vi "uber auto.vi"(1 "autobox switches":cluster{bool, bool, bool}) -> ()   [LabVIEW 2011]
uses:
  <vilib>/Rock Robotics/WPI/Solenoid/WPI_SolenoidValue.ctl
  <vilib>/addons/control/pid/pid.llb/PID (DBL).vi
  <vilib>/Rock Robotics/WPI/Solenoid/WPI_SolenoidSetEnum.vi
  <vilib>/Rock Robotics/WPI/Solenoid/Deprecated/WPI_SolenoidSetBool.vi
  <vilib>/addons/control/pid/NI_PID_pid.lvlib
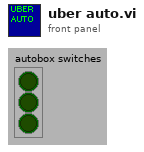
[diagram p1: front panel]
types:
  T1 = typedef "WPI_SolenoidDevRef.ctl" = cluster{"DevStatus":errorcluster, "Solenoid Module":T2, "Forward Solenoid Channel":T3, "Reverse Solenoid Channel":T3}
  T2 = typedef "FPGA_TypedefSolenoidModule.ctl" = enum16{"Solenoid Module 1", "Solenoid Module 2"}
  T3 = typedef "WPI_SolenoidChannel.ctl" = enum8{"Solenoid 1", "Solenoid 2", "Solenoid 3", "Solenoid 4", "Solenoid 5", "Solenoid 6", "Solenoid 7", "Solenoid 8", "Invalid"}
  T4 = typedef "WPI_EncoderDevRef.ctl" = cluster{"DevStatus":errorcluster, "EncoderIndex":T5, "CounterIndex":T6, "DistancePerCount":dbl, "Decoding Type":T7}
  T5 = typedef "FPGA_EncoderIdx.ctl" = enum8{"Enc 0", "Enc 1", "Enc 2", "Enc 3", "Invalid"}
  T6 = typedef "FPGA_CounterCtrSystemIndex.ctl" = enum8{"Ctr 0", "Ctr 1", "Ctr 2", "Ctr 3", "Ctr 4", "Ctr 5", "Ctr 6", "Ctr 7", "Invalid"}
  T7 = typedef "WPI_EncoderType.ctl" = enum16{"1x", "2x", "4x"}
  T8 = typedef "WPI_MotorControlDeviceRef.ctl" = cluster{"DeviceStatus":errorcluster, "Type":enum16{"PWM", "CAN"}, "PWM":cluster{"Digital Module":T9, "PWM Channel":T10, "DeadBand":T11}, "CAN":cluster{"Device Number":u8, "Control Mode":T12, "Semaphore":T13, "Max Vout":dbl}, "Invert":bool, "TransformRef":T14, "InvTransformRef":T14}
  T9 = typedef "FPGA_TypedefDigitalModule.ctl" = enum16{"Digital Module 1", "Digital Module 2"}
  T10 = typedef "FPGA_DIOPWMChannel.ctl" = enum8{"PWM 1", "PWM 2", "PWM 3", "PWM 4", "PWM 5", "PWM 6", "PWM 7", "PWM 8", "PWM 9", "PWM 10", "Invalid"}
  T11 = typedef "WPI_PWMDeadband.ctl" = cluster{"Name":string, "maxPositivePwm":i32, "minPositivePwm":i32, "centerPwm":i32, "maxNegativePwm":i32, "minNegativePwm":i32, "angularRange":u16}
  T12 = typedef "WPI_CANJaguar_ControlMode.ctl" = enum8{"Percent VBus", "Current", "Speed", "Position", "Voltage"}
  T13 = typedef "Semaphore RefNum" = refnum<k1>
  T14 = typedef "WPI_PWMTransform_ConPane.ctl" = refnum<vi>
  T15 = typedef "WPI_RobotDriveDevRef.ctl" = cluster{"DevStatus":errorcluster, "Motors[]":T8[], "Square Inputs":bool, "Max Output":dbl, "Isochronous":bool}
  T16 = cluster{"proportional gain (Kc)":dbl, "integral time (Ti, min)":dbl, "derivative time (Td, min)":dbl}
  T17 = typedef "WPI_SolenoidValue.ctl" = enum16{"Off", "On", "Forward", "Reverse"}
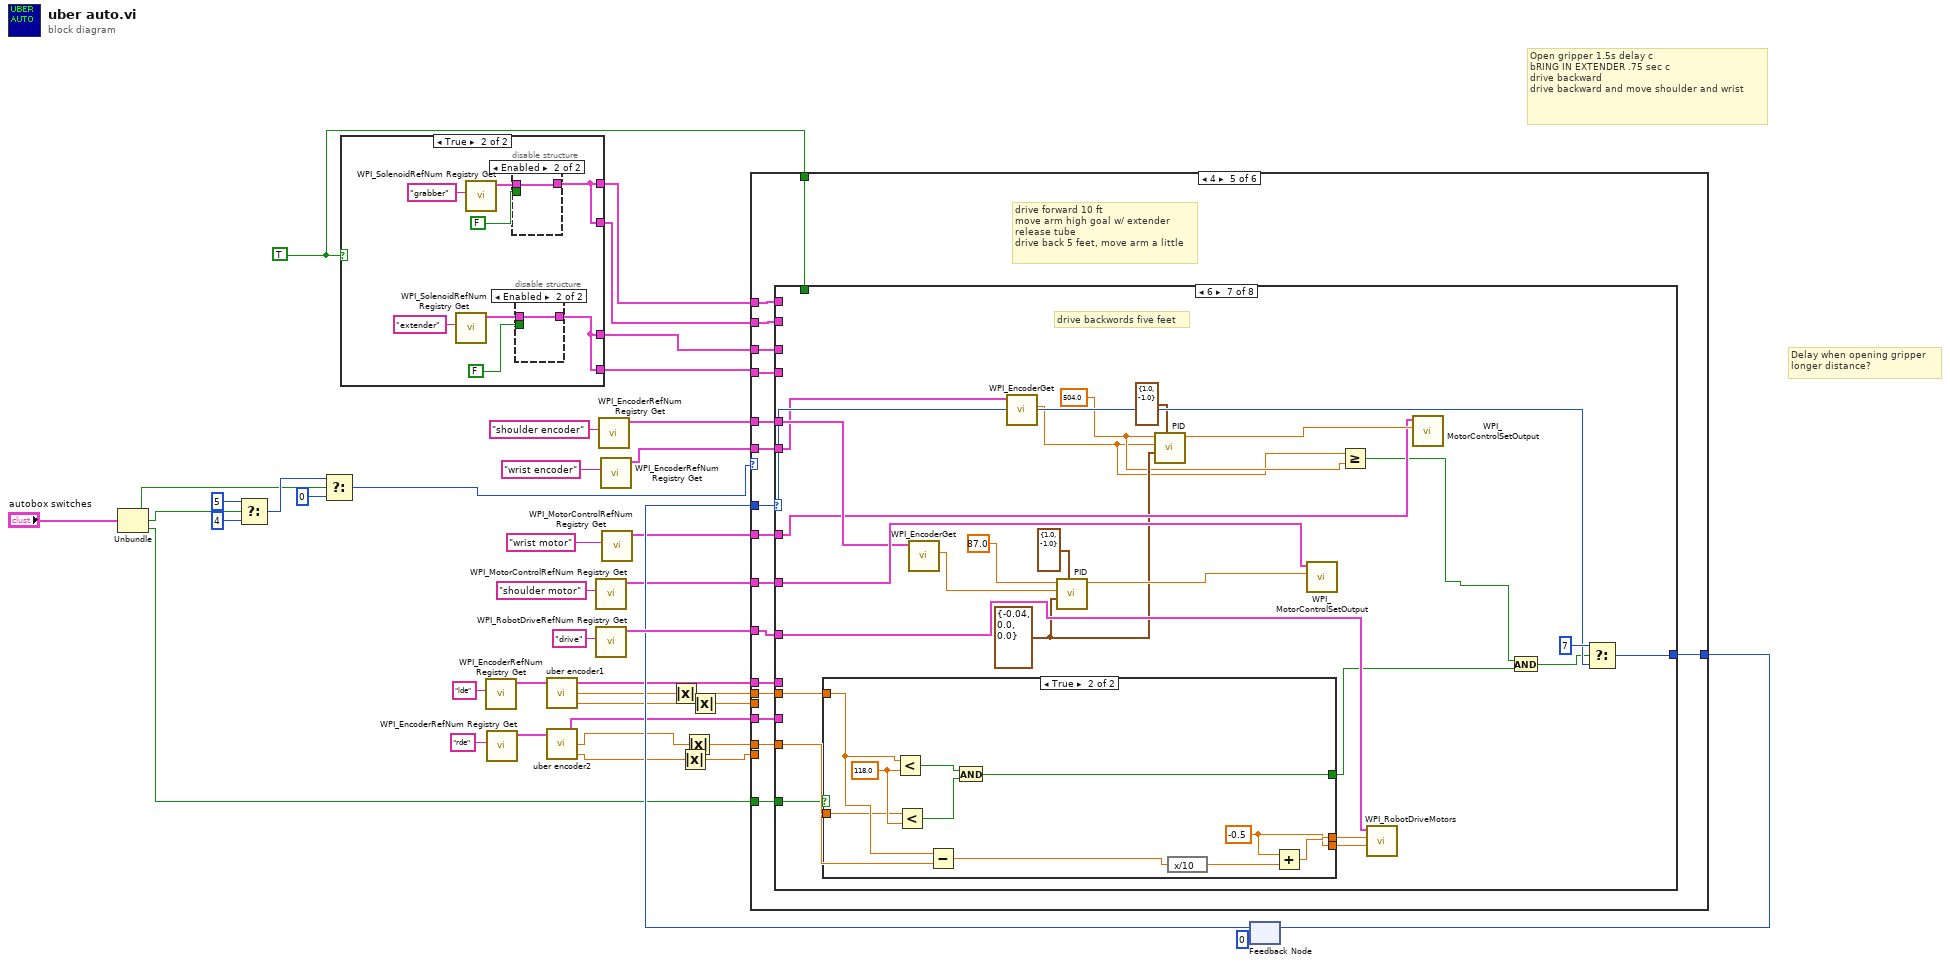
[diagram p0: block diagram]
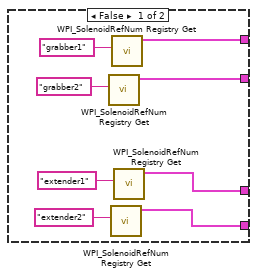
[diagram p2: hidden frame]
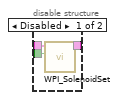
[diagram p3: hidden frame]
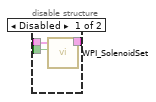
[diagram p4: hidden frame]
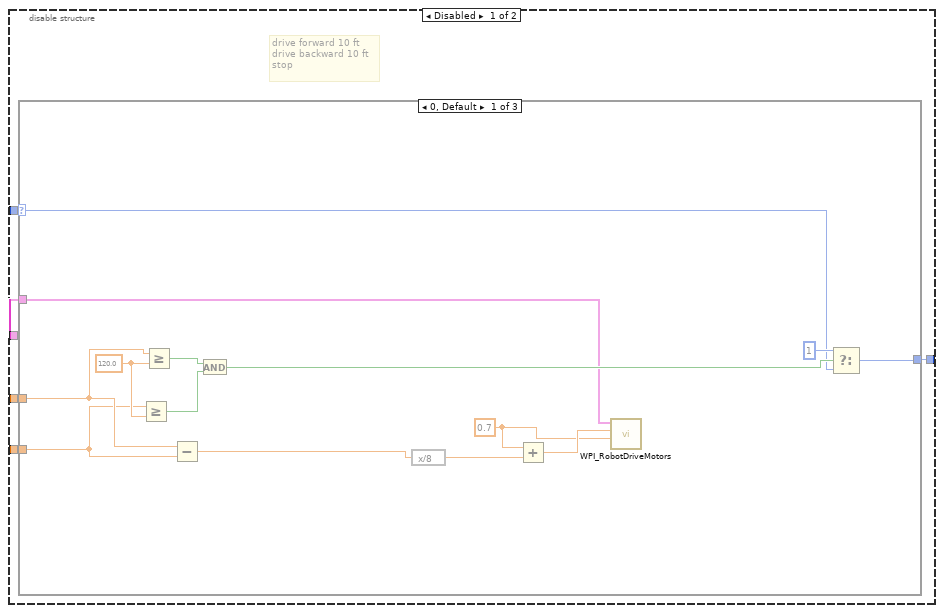
[diagram p6: hidden frame]
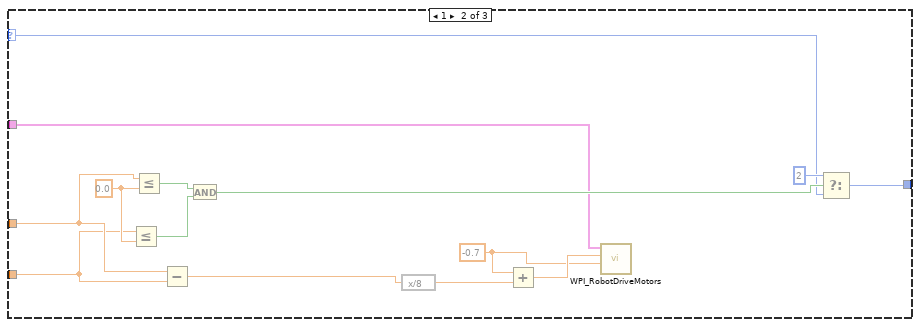
[diagram p7: hidden frame]
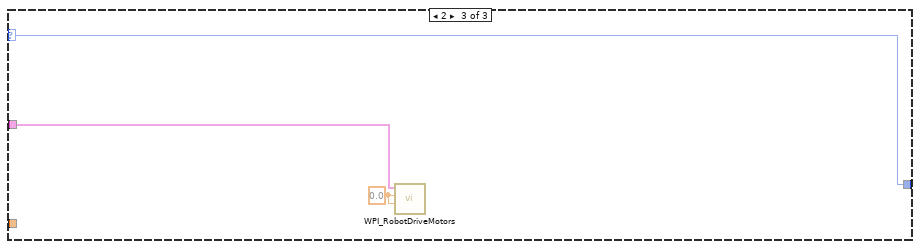
[diagram p8: hidden frame]
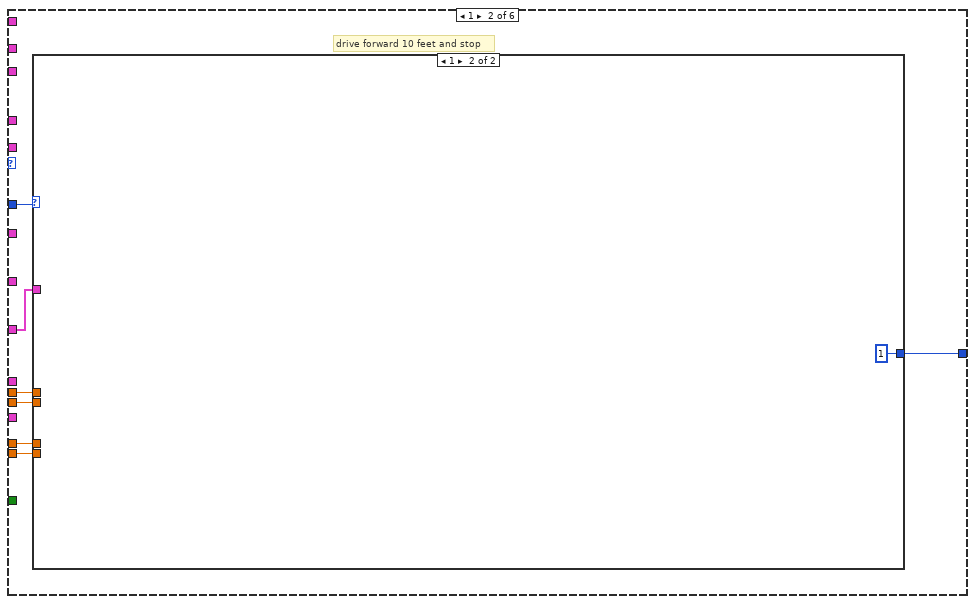
[diagram p9: hidden frame]
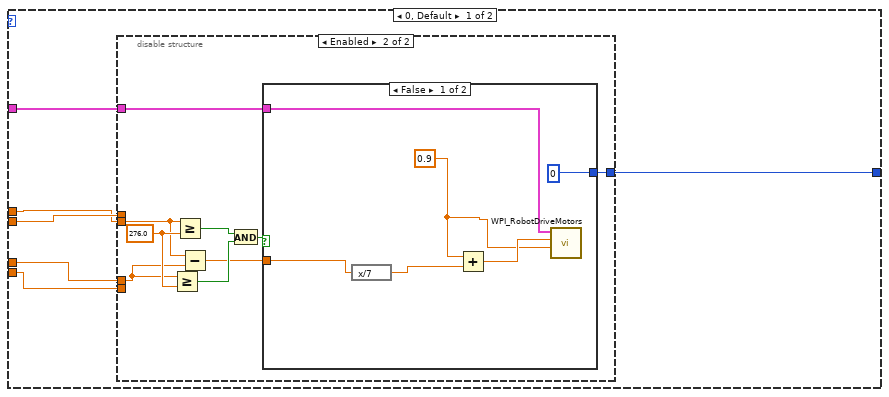
[diagram p10: hidden frame]
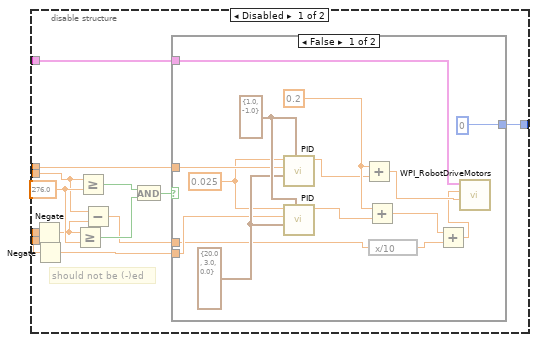
[diagram p11: hidden frame]
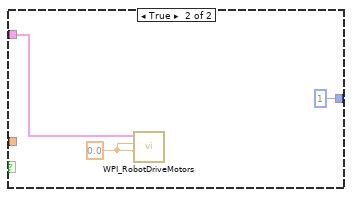
[diagram p12: hidden frame]
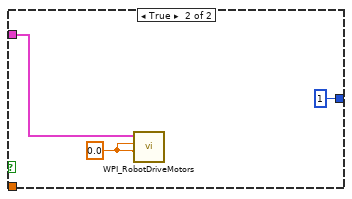
[diagram p13: hidden frame]
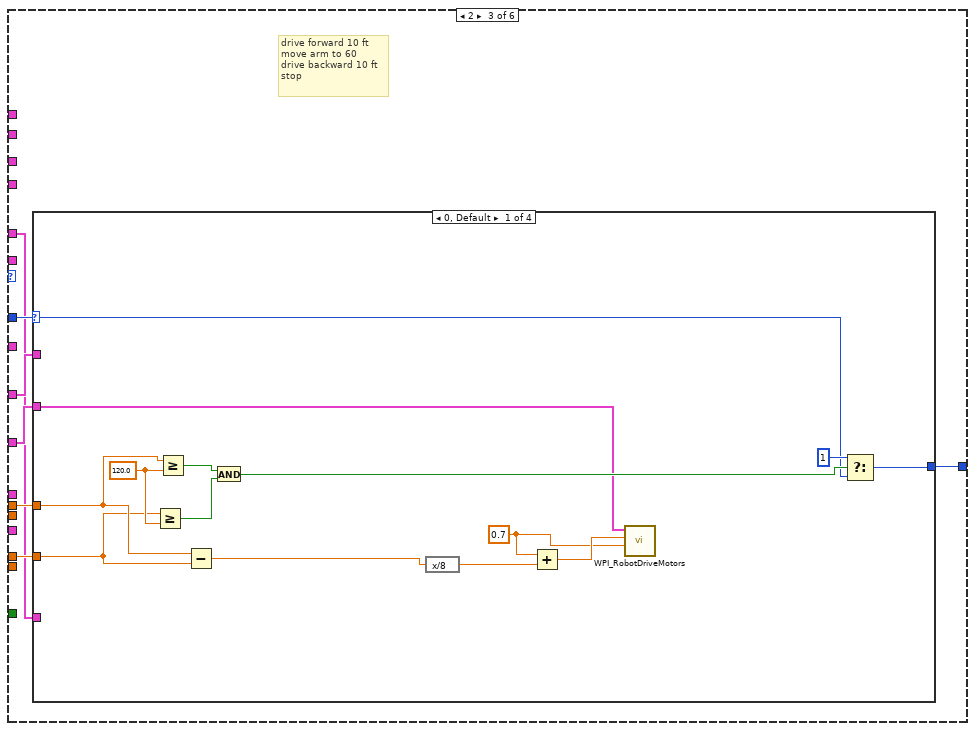
[diagram p14: hidden frame]
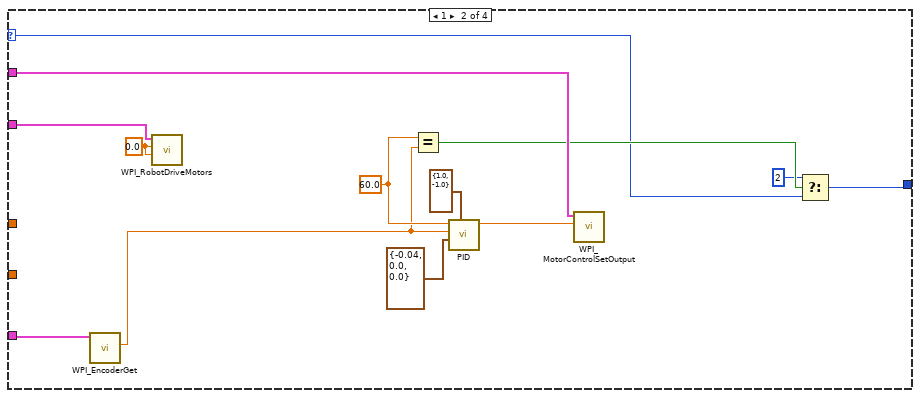
[diagram p15: hidden frame]
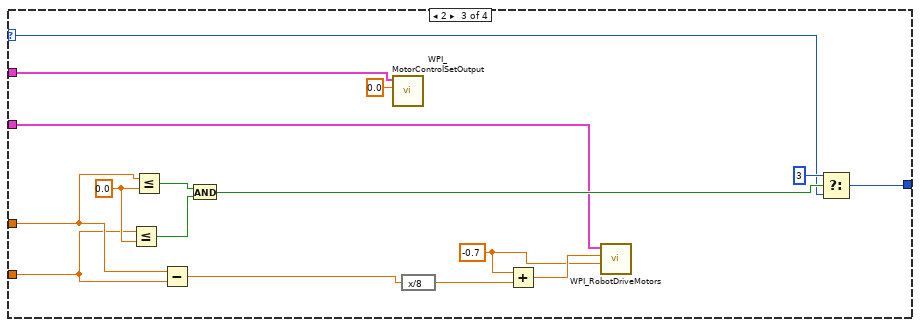
[diagram p16: hidden frame]
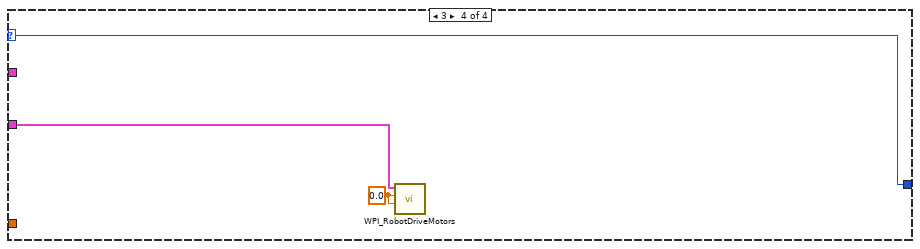
[diagram p17: hidden frame]
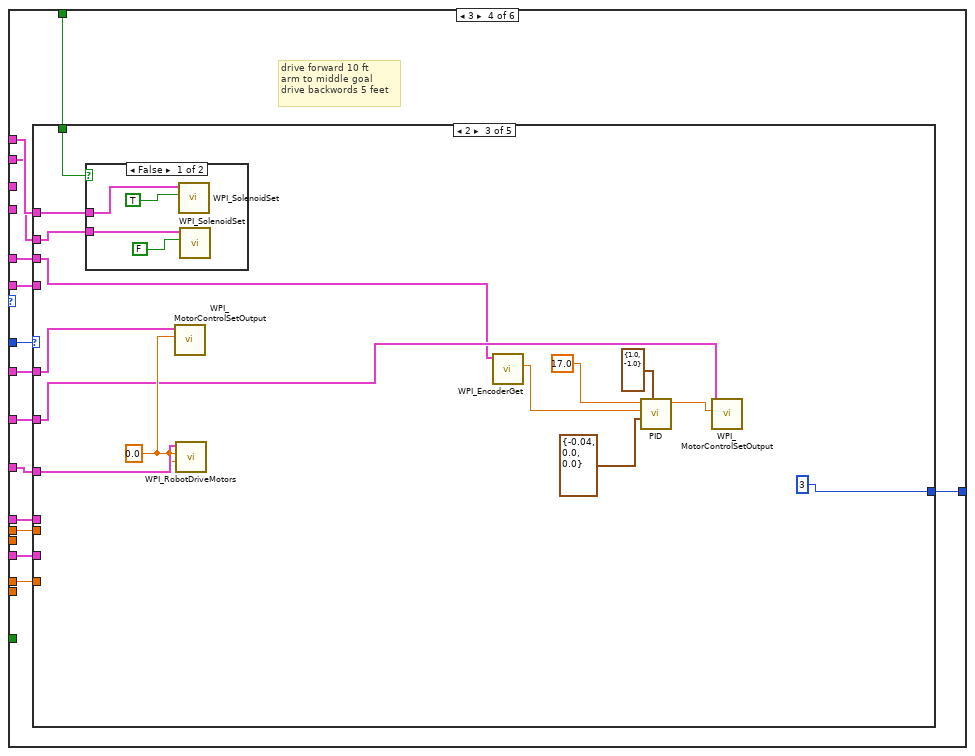
[diagram p18: hidden frame]
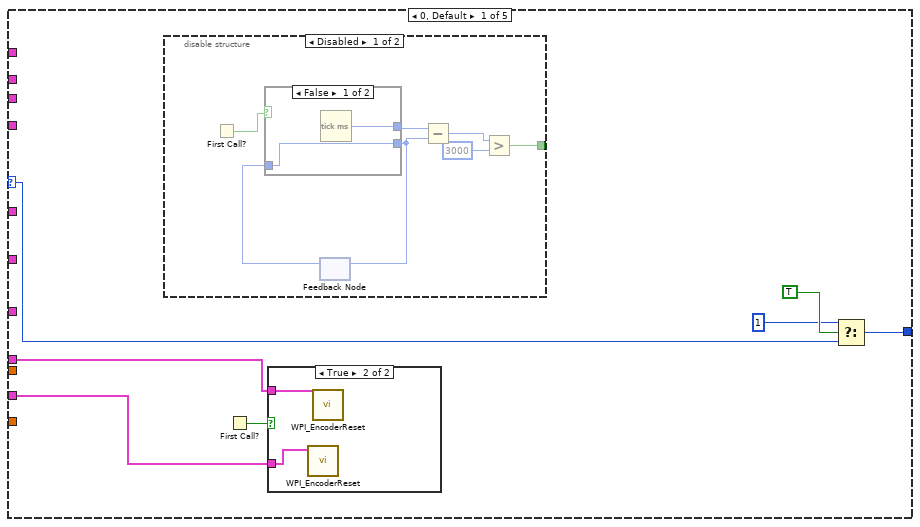
[diagram p19: hidden frame]
diagram:
  w1 = TRUE
  # "Open gripper 1.5s delay c\nbRING IN EXTENDER .75 sec c\ndrive backward\ndrive backward and move shoulder and wrist"
  # "Delay when opening gripper\nlonger distance?"
  n1 = Unbundle("autobox switches") -> (w16:bool, w19:bool, w13:bool)
  n2 = Select(t=5, s=w19, f=4) -> (s? t:f=w17:i32)
  n3 = Select(t=w17, s=w16, f=0) -> (s? t:f=w14:i32)
  n4 = case shown="True" w1 {
    tunnel: [w45 w51] -> w24
    tunnel: [w43 w50] -> w22
    tunnel: [w44 w51] -> w23
    tunnel: [w42 w50] -> w21
    frame False {
      n5 = call <vilib>:"WPI_SolenoidRefNum Registry Get.vi"("refnum name"="grabber2") -> ("SolenoidDevRef"=w44:T1)  [unwired: 1 in, 9 out]
      n6 = call <vilib>:"WPI_SolenoidRefNum Registry Get.vi"("refnum name"="extender2") -> ("SolenoidDevRef"=w42:T1)  [unwired: 1 in, 9 out]
      n7 = call <vilib>:"WPI_SolenoidRefNum Registry Get.vi"("refnum name"="grabber1") -> ("SolenoidDevRef"=w45:T1)  [unwired: 1 in, 9 out]
      n8 = call <vilib>:"WPI_SolenoidRefNum Registry Get.vi"("refnum name"="extender1") -> ("SolenoidDevRef"=w43:T1)  [unwired: 1 in, 9 out]
    }
    frame True {
      n9 = call <vilib>:"WPI_SolenoidRefNum Registry Get.vi"("refnum name"="extender") -> ("SolenoidDevRef"=w53:T1)  [unwired: 1 in, 9 out]
      n10 = call <vilib>:"WPI_SolenoidRefNum Registry Get.vi"("refnum name"="grabber") -> ("SolenoidDevRef"=w55:T1)  [unwired: 1 in, 9 out]
      n11 = disable-structure shown="Enabled" {
        disable-tunnel: w55 -> [w64 w65]
        disable-tunnel: FALSE ("Value") -> [w63 _]
        disable-tunnel: [w62 w65] -> w51
        frame Disabled {
          n12 = call-poly <vilib>:"WPI_SolenoidSet.vi"("Value"=w63, "SolenoidDevRef"=w64) -> ("SolenoidDevRef"=w62:T1)  [unwired: 1 in, 8 out]
        }
        frame Enabled {
        }
      }
      n13 = disable-structure shown="Enabled" {
        disable-tunnel: w53 -> [w60 w61]
        disable-tunnel: FALSE ("Value") -> [w59 _]
        disable-tunnel: [w58 w61] -> w50
        frame Disabled {
          n14 = call-poly <vilib>:"WPI_SolenoidSet.vi"("Value"=w59, "SolenoidDevRef"=w60) -> ("SolenoidDevRef"=w58:T1)  [unwired: 1 in, 8 out]
        }
        frame Enabled {
        }
      }
    }
  }
  n15 = call <vilib>:"WPI_EncoderRefNum Registry Get.vi"("refnum name"="lde") -> ("EncoderDevRef"=w33:T4)  [unwired: 1 in, 9 out]
  n16 = call <vilib>:"WPI_EncoderRefNum Registry Get.vi"("refnum name"="rde") -> ("EncoderDevRef"=w34:T4)  [unwired: 1 in, 9 out]
  n17 = call "uber encoder1.vi"("EncoderDevRef"=w33) -> ("rate"=w10:dbl, "Distance"=w11:dbl, "EncoderDevRef out"=w12:T4)  [unwired: 2 out]
  n18 = call "uber encoder2.vi"("EncoderDevRef"=w34) -> ("rate"=w7:dbl, "Distance"=w8:dbl, "EncoderDevRef out"=w9:T4)  [unwired: 2 out]
  n19 = call <vilib>:"WPI_MotorControlRefNum Registry Get.vi"("refnum name"="shoulder motor") -> ("MotorControlDevRef"=w30:T8)  [unwired: 1 in, 9 out]
  n20 = call <vilib>:"WPI_RobotDriveRefNum Registry Get.vi"("refnum name"="drive") -> ("RobotDriveDevRef"=w38:T15)  [unwired: 1 in, 9 out]
  n21 = call <vilib>:"WPI_EncoderRefNum Registry Get.vi"("refnum name"="shoulder encoder") -> ("EncoderDevRef"=w29:T4)  [unwired: 1 in, 9 out]
  n22 = call <vilib>:"WPI_EncoderRefNum Registry Get.vi"("refnum name"="wrist encoder") -> ("EncoderDevRef"=w26:T4)  [unwired: 1 in, 9 out]
  n23 = call <vilib>:"WPI_MotorControlRefNum Registry Get.vi"("refnum name"="wrist motor") -> ("MotorControlDevRef"=w25:T8)  [unwired: 1 in, 9 out]
  n24 = Absolute Value(x=w11) -> (abs(x)=w3:dbl)
  n25 = Absolute Value(x=w7) -> (abs(x)=w6:dbl)
  n26 = Absolute Value(x=w8) -> (abs(x)=w5:dbl)
  n27 = Absolute Value(x=w10) -> (abs(x)=w4:dbl)
  n28 = feedback #1(i64 0 ("state")) -> (w36:i64)
  n29 = case shown="4" w14 {
    tunnel: w36 -> [w66 w114 w173 w233 w366 w619]
    tunnel: w38 -> [w67 w113 w174 w234 w367 w620]
    tunnel: [w70 w112 w177 w237 w370 w623] -> w37
    tunnel: w3 -> [w69 w111 w176 w236 w369 w622]
    tunnel: w5 -> [w68 w110 w175 w235 w368 w621]
    tunnel: w6 -> [_ w109 _ _ _ _]
    tunnel: w4 -> [_ w108 _ _ _ _]
    tunnel: w30 -> [_ _ w172 w232 w365 w618]
    tunnel: w29 -> [_ _ w171 w231 w364 w617]
    tunnel: w26 -> [_ _ _ w230 w363 w616]
    tunnel: w25 -> [_ _ _ w229 w362 w615]
    tunnel: w24 -> [_ _ _ w228 w361 w614]
    tunnel: w23 -> [_ _ _ w227 w360 w613]
    tunnel: w1 -> [_ _ _ w226 w359 w612]
    tunnel: w22 -> [_ _ _ _ w358 w611]
    tunnel: w21 -> [_ _ _ _ w357 w610]
    tunnel: w12 -> [_ _ _ w225 w356 w609]
    tunnel: w9 -> [_ _ _ w224 w355 w608]
    tunnel: w13 -> [_ _ _ _ w354 w607]
    frame 0, Default {
      n30 = disable-structure shown="Enabled" {
        disable-tunnel: [w75 w107] -> w70
        disable-tunnel: w69 -> [w74 _]
        disable-tunnel: w68 -> [w73 _]
        disable-tunnel: w67 -> [w72 _]
        disable-tunnel: w66 -> [w71 w107]
        frame Disabled {
          # "drive forward 10 ft\ndrive backward 10 ft\nstop"
          n31 = case shown="0, Default" w71 {
            selector: w71 -> [w76 w90 w104]
            tunnel: [w89 w103 w104] -> w75
            tunnel: w74 -> [w83 w97 _]
            tunnel: w73 -> [w82 w96 _]
            tunnel: w72 -> [w77 w91 w106]
            frame 0, Default {
              w79 = 0.7 ("x")
              w85 = 120.0 ("y")
              n32 = Greater Or Equal?(x=w82, y=w85) -> (x >= y?=w86:bool)
              n33 = Greater Or Equal?(x=w83, y=w85) -> (x >= y?=w87:bool)
              n34 = Subtract(x=w83, y=w82) -> (x-y=w78:dbl)
              n35 = And(x=w87, y=w86) -> (x .and. y?=w84:bool)
              n36 = expression code="x/8"(w78) -> (w80:dbl)
              n37 = Add(x=w79, y=w80) -> (x+y=w81:dbl)
              n38 = call <vilib>:"WPI_RobotDriveMotors.vi"("RightSpeed"=w79, "LeftSpeed"=w81, "RobotDriveDevRef"=w77) -> ()  [unwired: 1 in, 8 out]
              n39 = Select(t=u32 1, s=w84, f=w76) -> (s? t:f=w89:i64)
            }
            frame 1 {
              w93 = -0.7 ("x")
              w99 = 0.0 ("y")
              n40 = Less Or Equal?(x=w96, y=w99) -> (x <= y?=w100:bool)
              n41 = Less Or Equal?(x=w97, y=w99) -> (x <= y?=w101:bool)
              n42 = Subtract(x=w97, y=w96) -> (x-y=w92:dbl)
              n43 = And(x=w101, y=w100) -> (x .and. y?=w98:bool)
              n44 = expression code="x/8"(w92) -> (w94:dbl)
              n45 = Add(x=w93, y=w94) -> (x+y=w95:dbl)
              n46 = call <vilib>:"WPI_RobotDriveMotors.vi"("RightSpeed"=w93, "LeftSpeed"=w95, "RobotDriveDevRef"=w91) -> ()  [unwired: 1 in, 8 out]
              n47 = Select(t=u32 2, s=w98, f=w90) -> (s? t:f=w103:i64)
            }
            frame 2 {
              w105 = 0.0 ("LeftSpeed")
              n48 = call <vilib>:"WPI_RobotDriveMotors.vi"("RightSpeed"=w105, "LeftSpeed"=w105, "RobotDriveDevRef"=w106) -> ()  [unwired: 1 in, 8 out]
            }
          }
        }
        frame Enabled {
          # "no autonomous"
        }
      }
    }
    frame 1 {
      # "drive forward 10 feet and stop"
      n49 = case shown="1" w114 {
        tunnel: w113 -> [w120 _]
        tunnel: [w119 u32 1 ("state")] -> w112
        tunnel: w111 -> [w117 _]
        tunnel: w110 -> [w116 _]
        tunnel: w109 -> [w115 _]
        tunnel: w108 -> [w118 _]
        frame 0, Default {
          n50 = disable-structure shown="Enabled" {
            disable-tunnel: w120 -> [w133 w159]
            disable-tunnel: [w128 w160] -> w119
            disable-tunnel: w118 -> [w127 _]
            disable-tunnel: w116 -> [w126 w152]
            disable-tunnel: w115 -> [w125 _]
            disable-tunnel: w117 -> [w123 w155]
            frame Disabled {
              w129 = 276.0 ("y")
              # "should not be (-)ed"
              n51 = Negate(x=w126) -> (-x=w122:dbl)
              n52 = Negate(x=w125) -> (-x=w124:dbl)
              n53 = Greater Or Equal?(x=w122, y=w129) -> (x >= y?=w130:bool)
              n54 = Greater Or Equal?(x=w123, y=w129) -> (x >= y?=w131:bool)
              n55 = Subtract(x=w123, y=w122) -> (x-y=w121:dbl)
              n56 = And(x=w131, y=w130) -> (x .and. y?=w132:bool)
              n57 = case shown="False" w132 {
                tunnel: w133 -> [w146 w151]
                tunnel: [u32 0 ("state") u32 1 ("state")] -> w128
                tunnel: w127 -> [w144 _]
                tunnel: w124 -> [w143 _]
                tunnel: w121 -> [w137 _]
                frame False {
                  w147 = T16 {"proportional gain (Kc)"=20.0, "integral time (Ti, min)"=3.0, "derivative time (Td, min)"=0.0} ("PID gains")
                  w148 = cluster{"output high":dbl, "output low":dbl} {"output high"=1.0, "output low"=-1.0} ("output range")
                  w141 = 0.2 ("setpoint")
                  w142 = 0.025 ("setpoint")
                  n58 = call-poly <vilib>:"PID.vi"("output range"=w148, "PID gains"=w147, "process variable"=w144, "setpoint"=w142) -> ("output"=w139:dbl)  [unwired: 2 in, 5 out]
                  n59 = call-poly <vilib>:"PID.vi"("output range"=w148, "PID gains"=w147, "process variable"=w143, "setpoint"=w142) -> ("output"=w140:dbl)  [unwired: 2 in, 5 out]
                  n60 = Add(x=w141, y=w139) -> (x+y=w138:dbl)
                  n61 = Add(x=w141, y=w140) -> (x+y=w135:dbl)
                  n62 = expression code="x/10"(w137) -> (w136:dbl)
                  n63 = Add(x=w135, y=w136) -> (x+y=w134:dbl)
                  n64 = call <vilib>:"WPI_RobotDriveMotors.vi"("RightSpeed"=w138, "LeftSpeed"=w134, "RobotDriveDevRef"=w146) -> ()  [unwired: 1 in, 8 out]
                }
                frame True {
                  w150 = 0.0 ("LeftSpeed")
                  n65 = call <vilib>:"WPI_RobotDriveMotors.vi"("RightSpeed"=w150, "LeftSpeed"=w150, "RobotDriveDevRef"=w151) -> ()  [unwired: 1 in, 8 out]
                }
              }
            }
            frame Enabled {
              w158 = 276.0 ("y")
              n66 = Greater Or Equal?(x=w152, y=w158) -> (x >= y?=w157:bool)
              n67 = Greater Or Equal?(x=w155, y=w158) -> (x >= y?=w156:bool)
              n68 = Subtract(x=w155, y=w152) -> (x-y=w154:dbl)
              n69 = And(x=w156, y=w157) -> (x .and. y?=w153:bool)
              n70 = case shown="False" w153 {
                tunnel: w159 -> [w166 w169]
                tunnel: [u32 0 ("state") u32 1 ("state")] -> w160
                tunnel: w154 -> [w163 _]
                frame False {
                  w161 = 0.9 ("x")
                  n71 = expression code="x/7"(w163) -> (w162:dbl)
                  n72 = Add(x=w161, y=w162) -> (x+y=w164:dbl)
                  n73 = call <vilib>:"WPI_RobotDriveMotors.vi"("RightSpeed"=w161, "LeftSpeed"=w164, "RobotDriveDevRef"=w166) -> ()  [unwired: 1 in, 8 out]
                }
                frame True {
                  w168 = 0.0 ("LeftSpeed")
                  n74 = call <vilib>:"WPI_RobotDriveMotors.vi"("RightSpeed"=w168, "LeftSpeed"=w168, "RobotDriveDevRef"=w169) -> ()  [unwired: 1 in, 8 out]
                }
              }
            }
          }
        }
        frame 1 {
        }
      }
    }
    frame 2 {
      # "drive forward 10 ft\nmove arm to 60\ndrive backward 10 ft\nstop"
      n75 = case shown="0, Default" w173 {
        selector: w173 -> [w178 w195 w207 w221]
        tunnel: [w191 w196 w220 w221] -> w177
        tunnel: w176 -> [w185 _ w214 _]
        tunnel: w175 -> [w184 _ w213 _]
        tunnel: w174 -> [w179 w193 w208 w223]
        tunnel: w172 -> [_ w201 w206 _]
        tunnel: w171 -> [_ w202 _ _]
        frame 0, Default {
          w181 = 0.7 ("x")
          w187 = 120.0 ("y")
          n76 = Greater Or Equal?(x=w184, y=w187) -> (x >= y?=w188:bool)
          n77 = Greater Or Equal?(x=w185, y=w187) -> (x >= y?=w189:bool)
          n78 = Subtract(x=w185, y=w184) -> (x-y=w180:dbl)
          n79 = And(x=w189, y=w188) -> (x .and. y?=w186:bool)
          n80 = expression code="x/8"(w180) -> (w182:dbl)
          n81 = Add(x=w181, y=w182) -> (x+y=w183:dbl)
          n82 = call <vilib>:"WPI_RobotDriveMotors.vi"("RightSpeed"=w181, "LeftSpeed"=w183, "RobotDriveDevRef"=w179) -> ()  [unwired: 1 in, 8 out]
          n83 = Select(t=u32 1, s=w186, f=w178) -> (s? t:f=w191:i64)
        }
        frame 1 {
          w192 = 0.0 ("LeftSpeed")
          w199 = 60.0 ("setpoint")
          n84 = call <vilib>:"WPI_EncoderGet.vi"("EncoderDevRef"=w202) -> ("Distance"=w198:dbl)  [unwired: 1 in, 9 out]
          n85 = call <vilib>:"WPI_RobotDriveMotors.vi"("RightSpeed"=w192, "LeftSpeed"=w192, "RobotDriveDevRef"=w193) -> ()  [unwired: 1 in, 8 out]
          n86 = Equal?(x=w199, y=w198) -> (x = y?=w197:bool)
          n87 = call-poly <vilib>:"PID.vi"("output range"=cluster{"output high":dbl, "output low":dbl} {"output high"=1.0, "output low"=-1.0}, "PID gains"=T16 {"proportional gain (Kc)"=-0.04, "integral time (Ti, min)"=0.0, "derivative time (Td, min)"=0.0}, "process variable"=w198, "setpoint"=w199) -> ("output"=w200:dbl)  [unwired: 3 in, 4 out]
          n88 = call <vilib>:"WPI_MotorControlSetOutput.vi"("Output"=w200, "MotorControlDevRef"=w201) -> ()  [unwired: 3 in, 7 out]
          n89 = Select(t=u32 2, s=w197, f=w195) -> (s? t:f=w196:i64)
        }
        frame 2 {
          w210 = -0.7 ("x")
          w216 = 0.0 ("y")
          n90 = Less Or Equal?(x=w213, y=w216) -> (x <= y?=w217:bool)
          n91 = Less Or Equal?(x=w214, y=w216) -> (x <= y?=w218:bool)
          n92 = Subtract(x=w214, y=w213) -> (x-y=w209:dbl)
          n93 = And(x=w218, y=w217) -> (x .and. y?=w215:bool)
          n94 = call <vilib>:"WPI_MotorControlSetOutput.vi"("Output"=0.0, "MotorControlDevRef"=w206) -> ()  [unwired: 3 in, 7 out]
          n95 = expression code="x/8"(w209) -> (w211:dbl)
          n96 = Add(x=w210, y=w211) -> (x+y=w212:dbl)
          n97 = call <vilib>:"WPI_RobotDriveMotors.vi"("RightSpeed"=w210, "LeftSpeed"=w212, "RobotDriveDevRef"=w208) -> ()  [unwired: 1 in, 8 out]
          n98 = Select(t=u32 3, s=w215, f=w207) -> (s? t:f=w220:i64)
        }
        frame 3 {
          w222 = 0.0 ("LeftSpeed")
          n99 = call <vilib>:"WPI_RobotDriveMotors.vi"("RightSpeed"=w222, "LeftSpeed"=w222, "RobotDriveDevRef"=w223) -> ()  [unwired: 1 in, 8 out]
        }
      }
    }
    frame 3 {
      # "drive forward 10 ft\narm to middle goal\ndrive backwords 5 feet"
      n100 = case shown="2" w233 {
        selector: w233 -> [w243 w272 _ w321 w345]
        tunnel: [w244 w285 u32 3 ("t") w334 w345] -> w237
        tunnel: w236 -> [_ w279 _ w328 _]
        tunnel: w235 -> [_ w278 _ w327 _]
        tunnel: w234 -> [_ w273 w307 w322 w347]
        tunnel: w232 -> [_ w268 w295 w315 w336]
        tunnel: w231 -> [_ w267 w294 w314 w335]
        tunnel: w230 -> [_ w259 _ _ _]
        tunnel: w229 -> [_ w261 w306 _ _]
        tunnel: w228 -> [_ _ w303 _ w344]
        tunnel: w227 -> [_ _ w302 _ w343]
        tunnel: w226 -> [_ _ w301 _ w342]
        tunnel: w225 -> [w239 _ _ _ _]
        tunnel: w224 -> [w238 _ _ _ _]
        frame 0, Default {
          n101 = disable-structure shown="Disabled" {
            disable-tunnel: [w247 _] -> _
            frame Disabled {
              n102 = First Call?() -> (First Call?: T/F=w253:bool)
              n103 = feedback #2() -> (w252:u32)  [unwired: 1 out]
              n104 = case shown="False" w253 {
                tunnel: [w255 w256] -> w250
                tunnel: w252 -> [w255 _]
                tunnel: [w254 w256] -> w251
                frame False {
                  n105 = Tick Count (ms)() -> (millisecond timer value=w254:u32)
                }
                frame True {
                  n106 = Tick Count (ms)() -> (millisecond timer value=w256:u32)
                }
              }
              n107 = feedback-in #2(w250) -> ()
              n108 = Subtract(x=w251, y=w250) -> (x-y=w249:u32)
              n109 = Greater?(x=w249, y=u32 3000) -> (0:w247:bool)
            }
            frame Enabled {
            }
          }
          n110 = First Call?() -> (First Call?: T/F=w240:bool)
          n111 = case shown="True" w240 {
            tunnel: w239 -> [_ w246]
            tunnel: w238 -> [_ w245]
            frame False {
            }
            frame True {
              n112 = call <vilib>:"WPI_EncoderReset.vi"("EncoderDevRef"=w245) -> ()  [unwired: 1 in, 10 out]
              n113 = call <vilib>:"WPI_EncoderReset.vi"("EncoderDevRef"=w246) -> ()  [unwired: 1 in, 10 out]
            }
          }
          n114 = Select(t=u32 1, s=TRUE, f=w243) -> (s? t:f=w244:i64)
        }
        frame 1 {
          w260 = T16 {"proportional gain (Kc)"=-0.04, "integral time (Ti, min)"=0.0, "derivative time (Td, min)"=0.0} ("PID gains")
          w262 = 276.0 ("setpoint")
          w271 = 17.0 ("setpoint")
          w275 = 0.7 ("x")
          w281 = 156.0 ("y")
          n115 = Greater Or Equal?(x=w279, y=w281) -> (x >= y?=w283:bool)
          n116 = Greater Or Equal?(x=w278, y=w281) -> (x >= y?=w282:bool)
          n117 = call <vilib>:"WPI_EncoderGet.vi"("EncoderDevRef"=w267) -> ("Distance"=w266:dbl)  [unwired: 1 in, 9 out]
          n118 = Subtract(x=w279, y=w278) -> (x-y=w274:dbl)
          n119 = And(x=w283, y=w282) -> (x .and. y?=w280:bool)
          n120 = call <vilib>:"WPI_EncoderGet.vi"("EncoderDevRef"=w259) -> ("Distance"=w265:dbl)  [unwired: 1 in, 9 out]
          n121 = Equal?(x=w271, y=w266) -> (x = y?=w258:bool)
          n122 = call-poly <vilib>:"PID.vi"("output range"=cluster{"output high":dbl, "output low":dbl} {"output high"=1.0, "output low"=-1.0}, "PID gains"=w260, "process variable"=w266, "setpoint"=w271) -> ("output"=w270:dbl)  [unwired: 3 in, 4 out]
          n123 = Equal?(x=w262, y=w265) -> (x = y?=w257:bool)
          n124 = call-poly <vilib>:"PID.vi"("output range"=cluster{"output high":dbl, "output low":dbl} {"output high"=1.0, "output low"=-1.0}, "PID gains"=w260, "process variable"=w265, "setpoint"=w262) -> ("output"=w263:dbl)  [unwired: 3 in, 4 out]
          n125 = expression code="x/8"(w274) -> (w276:dbl)
          n126 = Add(x=w275, y=w276) -> (x+y=w277:dbl)
          n127 = case shown="False" w258 {
            tunnel: w270 -> [w291 _]
            tunnel: w268 -> [w290 w292]
            frame False {
              n128 = call <vilib>:"WPI_MotorControlSetOutput.vi"("Output"=w291, "MotorControlDevRef"=w290) -> ()  [unwired: 3 in, 7 out]
            }
            frame True {
              n129 = call <vilib>:"WPI_MotorControlSetOutput.vi"("Output"=0.0, "MotorControlDevRef"=w292) -> ()  [unwired: 3 in, 7 out]
            }
          }
          n130 = call <vilib>:"WPI_RobotDriveMotors.vi"("RightSpeed"=w275, "LeftSpeed"=w277, "RobotDriveDevRef"=w273) -> ()  [unwired: 1 in, 8 out]
          n131 = case shown="False" w257 {
            tunnel: w263 -> [_ w288]
            tunnel: w261 -> [w287 w289]
            frame True {
              n132 = call <vilib>:"WPI_MotorControlSetOutput.vi"("Output"=0.0, "MotorControlDevRef"=w287) -> ()  [unwired: 3 in, 7 out]
            }
            frame False {
              n133 = call <vilib>:"WPI_MotorControlSetOutput.vi"("Output"=w288, "MotorControlDevRef"=w289) -> ()  [unwired: 3 in, 7 out]
            }
          }
          n134 = Select(t=u32 2, s=w280, f=w272) -> (s? t:f=w285:i64)
        }
        frame 2 {
          w305 = 0.0 ("LeftSpeed")
          n135 = case shown="False" w301 {
            tunnel: w303 -> [w309 w313]
            tunnel: w302 -> [w308 _]
            frame False {
              n136 = call-poly <vilib>:"WPI_SolenoidSet.vi"("Value"=TRUE, "SolenoidDevRef"=w309) -> ()  [unwired: 1 in, 9 out]
              n137 = call-poly <vilib>:"WPI_SolenoidSet.vi"("Value"=FALSE, "SolenoidDevRef"=w308) -> ()  [unwired: 1 in, 9 out]
            }
            frame True {
              n138 = call-poly <vilib>:"WPI_SolenoidSet.vi"("Value"=WPI_SolenoidValue."On", "SolenoidDevRef"=w313) -> ()  [unwired: 1 in, 9 out]
            }
          }
          n139 = call <vilib>:"WPI_MotorControlSetOutput.vi"("Output"=w305, "MotorControlDevRef"=w306) -> ()  [unwired: 3 in, 7 out]
          n140 = call <vilib>:"WPI_RobotDriveMotors.vi"("RightSpeed"=w305, "LeftSpeed"=w305, "RobotDriveDevRef"=w307) -> ()  [unwired: 1 in, 8 out]
          n141 = call <vilib>:"WPI_EncoderGet.vi"("EncoderDevRef"=w294) -> ("Distance"=w298:dbl)  [unwired: 1 in, 9 out]
          n142 = call-poly <vilib>:"PID.vi"("output range"=cluster{"output high":dbl, "output low":dbl} {"output high"=1.0, "output low"=-1.0}, "PID gains"=T16 {"proportional gain (Kc)"=-0.04, "integral time (Ti, min)"=0.0, "derivative time (Td, min)"=0.0}, "process variable"=w298, "setpoint"=17.0) -> ("output"=w300:dbl)  [unwired: 3 in, 4 out]
          n143 = call <vilib>:"WPI_MotorControlSetOutput.vi"("Output"=w300, "MotorControlDevRef"=w295) -> ()  [unwired: 3 in, 7 out]
        }
        frame 3 {
          w324 = -0.7 ("x")
          w330 = 60.0 ("y")
          n144 = Less Or Equal?(x=w327, y=w330) -> (x <= y?=w331:bool)
          n145 = Less Or Equal?(x=w328, y=w330) -> (x <= y?=w332:bool)
          n146 = Subtract(x=w328, y=w327) -> (x-y=w323:dbl)
          n147 = And(x=w332, y=w331) -> (x .and. y?=w329:bool)
          n148 = expression code="x/8"(w323) -> (w325:dbl)
          n149 = call <vilib>:"WPI_EncoderGet.vi"("EncoderDevRef"=w314) -> ("Distance"=w318:dbl)  [unwired: 1 in, 9 out]
          n150 = Add(x=w324, y=w325) -> (x+y=w326:dbl)
          n151 = call-poly <vilib>:"PID.vi"("output range"=cluster{"output high":dbl, "output low":dbl} {"output high"=1.0, "output low"=-1.0}, "PID gains"=T16 {"proportional gain (Kc)"=-0.04, "integral time (Ti, min)"=0.0, "derivative time (Td, min)"=0.0}, "process variable"=w318, "setpoint"=17.0) -> ("output"=w316:dbl)  [unwired: 3 in, 4 out]
          n152 = call <vilib>:"WPI_RobotDriveMotors.vi"("RightSpeed"=w324, "LeftSpeed"=w326, "RobotDriveDevRef"=w322) -> ()  [unwired: 1 in, 8 out]
          n153 = call <vilib>:"WPI_MotorControlSetOutput.vi"("Output"=w316, "MotorControlDevRef"=w315) -> ()  [unwired: 3 in, 7 out]
          n154 = Select(t=u32 4, s=w329, f=w321) -> (s? t:f=w334:i64)
        }
        frame 4 {
          w346 = 0.0 ("LeftSpeed")
          n155 = case shown="False" w342 {
            tunnel: w344 -> [w349 _]
            tunnel: w343 -> [w348 w353]
            frame False {
              n156 = call-poly <vilib>:"WPI_SolenoidSet.vi"("Value"=FALSE, "SolenoidDevRef"=w349) -> ()  [unwired: 1 in, 9 out]
              n157 = call-poly <vilib>:"WPI_SolenoidSet.vi"("Value"=TRUE, "SolenoidDevRef"=w348) -> ()  [unwired: 1 in, 9 out]
            }
            frame True {
              n158 = call-poly <vilib>:"WPI_SolenoidSet.vi"("Value"=WPI_SolenoidValue."Off", "SolenoidDevRef"=w353) -> ()  [unwired: 1 in, 9 out]
            }
          }
          n159 = call <vilib>:"WPI_RobotDriveMotors.vi"("RightSpeed"=w346, "LeftSpeed"=w346, "RobotDriveDevRef"=w347) -> ()  [unwired: 1 in, 8 out]
          n160 = call <vilib>:"WPI_EncoderGet.vi"("EncoderDevRef"=w335) -> ("Distance"=w339:dbl)  [unwired: 1 in, 9 out]
          n161 = call-poly <vilib>:"PID.vi"("output range"=cluster{"output high":dbl, "output low":dbl} {"output high"=1.0, "output low"=-1.0}, "PID gains"=T16 {"proportional gain (Kc)"=-0.04, "integral time (Ti, min)"=0.0, "derivative time (Td, min)"=0.0}, "process variable"=w339, "setpoint"=17.0) -> ("output"=w337:dbl)  [unwired: 3 in, 4 out]
          n162 = call <vilib>:"WPI_MotorControlSetOutput.vi"("Output"=w337, "MotorControlDevRef"=w336) -> ()  [unwired: 3 in, 7 out]
        }
      }
    }
    frame 4 {
      # "drive forward 10 ft\nmove arm high goal w/ extender\nrelease tube\ndrive back 5 feet, move arm a little"
      n163 = case shown="6" w366 {
        selector: w366 -> [w376 w389 w417 _ w484 w514 w564 _]
        tunnel: [w377 w410 w420 u32 4 ("t") w492 w513 w571 u32 7 ("t")] -> w370
        tunnel: w369 -> [_ w405 w423 _ w488 _ w569 _]
        tunnel: w368 -> [_ w404 w422 _ w487 _ w568 _]
        tunnel: w367 -> [_ w399 w421 w464 w485 w526 w565 w598]
        tunnel: w365 -> [_ _ w431 w451 w478 w516 w561 w585]
        tunnel: w364 -> [_ _ w434 w454 w477 w515 w560 w588]
        tunnel: w363 -> [_ _ w435 _ _ _ w555 _]
        tunnel: w362 -> [_ _ w432 w463 _ _ w557 w597]
        tunnel: w361 -> [_ _ _ w460 w475 _ _ w594]
        tunnel: w360 -> [_ _ _ w459 w474 _ _ w593]
        tunnel: w359 -> [_ _ w416 w458 w476 w524 _ w592]
        tunnel: w358 -> [_ _ w415 _ _ w523 _ _]
        tunnel: w357 -> [_ _ w414 _ w473 w522 _ w584]
        tunnel: w356 -> [w372 _ _ _ _ _ _ _]
        tunnel: w355 -> [w371 _ _ _ _ _ _ _]
        tunnel: w354 -> [_ _ _ _ _ _ w554 _]
        frame 0, Default {
          # "reset encoders"
          n164 = disable-structure shown="Disabled" {
            disable-tunnel: [w380 _] -> _
            frame Disabled {
              n165 = feedback #3() -> (w385:u32)  [unwired: 1 out]
              n166 = case shown="False" {
                selector: _ -> [_ _]
                tunnel: [w387 w388] -> w383
                tunnel: w385 -> [w387 _]
                tunnel: [w386 w388] -> w384
                frame False {
                  n167 = Tick Count (ms)() -> (millisecond timer value=w386:u32)
                }
                frame True {
                  n168 = Tick Count (ms)() -> (millisecond timer value=w388:u32)
                }
              }
              n169 = feedback-in #3(w383) -> ()
              n170 = Subtract(x=w384, y=w383) -> (x-y=w382:u32)
              n171 = Greater?(x=w382, y=u32 3000) -> (0:w380:bool)
            }
            frame Enabled {
            }
          }
          n172 = First Call?() -> (First Call?: T/F=w373:bool)
          n173 = case shown="True" w373 {
            tunnel: w372 -> [_ w379]
            tunnel: w371 -> [_ w378]
            frame False {
            }
            frame True {
              n174 = call <vilib>:"WPI_EncoderReset.vi"("EncoderDevRef"=w378) -> ()  [unwired: 1 in, 10 out]
              n175 = call <vilib>:"WPI_EncoderReset.vi"("EncoderDevRef"=w379) -> ()  [unwired: 1 in, 10 out]
            }
          }
          n176 = Select(t=i64 1, s=TRUE, f=w376) -> (s? t:f=w377:i64)
        }
        frame 1 {
          w401 = 0.7 ("x")
          w406 = 178.0 ("y")
          # "x"
          # "Starts driving"
          # "drive forward 170 inches, advance after 1.5 seconds"
          n177 = Greater Or Equal?(x=w405, y=w406) -> (x >= y?=w408:bool)
          n178 = Greater Or Equal?(x=w404, y=w406) -> (x >= y?=w407:bool)
          n179 = Subtract(x=w405, y=w404) -> (x-y=w400:dbl)
          n180 = And(x=w408, y=w407) -> (x .and. y?=w393:bool)
          n181 = expression code="x/8"(w400) -> (w402:dbl)
          n182 = First Call?() -> (First Call?: T/F=w390:bool)
          n183 = Add(x=w401, y=w402) -> (x+y=w403:dbl)
          n184 = feedback #4() -> (w394:u32)  [unwired: 1 out]
          n185 = case shown="False" w390 {
            tunnel: [w412 w413] -> w396
            tunnel: w394 -> [w412 _]
            tunnel: [w411 w413] -> w395
            frame False {
              n186 = Tick Count (ms)() -> (millisecond timer value=w411:u32)
            }
            frame True {
              n187 = Tick Count (ms)() -> (millisecond timer value=w413:u32)
            }
          }
          n188 = feedback-in #4(w396) -> ()
          n189 = call <vilib>:"WPI_RobotDriveMotors.vi"("RightSpeed"=w401, "LeftSpeed"=w403, "RobotDriveDevRef"=w399) -> ()  [unwired: 1 in, 8 out]
          n190 = Subtract(x=w395, y=w396) -> (x-y=w397:u32)
          n191 = Greater?(x=w397, y=u32 1500) -> (0:w392:bool)
          n192 = Or(x=w392, y=w393) -> (x .or. y?=w391:bool)
          n193 = Select(t=i64 2, s=w391, f=w389) -> (s? t:f=w410:i64)
        }
        frame 2 {
          w433 = T16 {"proportional gain (Kc)"=-0.04, "integral time (Ti, min)"=0.0, "derivative time (Td, min)"=0.0} ("PID gains")
          w429 = 0.7 ("x")
          w426 = 178.0 ("y")
          # "x"
          # "drive 170 inches, move arm to high position, extend extender"
          n194 = case shown="True" w416 {
            tunnel: w415 -> [w446 w449]
            tunnel: w414 -> [w447 _]
            frame False {
              n195 = call-poly <vilib>:"WPI_SolenoidSet.vi"("Value"=TRUE, "SolenoidDevRef"=w446) -> ()  [unwired: 1 in, 9 out]
              n196 = call-poly <vilib>:"WPI_SolenoidSet.vi"("Value"=FALSE, "SolenoidDevRef"=w447) -> ()  [unwired: 1 in, 9 out]
            }
            frame True {
              n197 = call-poly <vilib>:"WPI_SolenoidSet.vi"("Value"=TRUE, "SolenoidDevRef"=w449) -> ()  [unwired: 1 in, 9 out]
            }
          }
          n198 = Greater Or Equal?(x=w423, y=w426) -> (x >= y?=w424:bool)
          n199 = Greater Or Equal?(x=w422, y=w426) -> (x >= y?=w425:bool)
          n200 = call <vilib>:"WPI_EncoderGet.vi"("EncoderDevRef"=w434) -> ("Distance"=w439:dbl)  [unwired: 1 in, 9 out]
          n201 = Subtract(x=w423, y=w422) -> (x-y=w430:dbl)
          n202 = And(x=w424, y=w425) -> (x .and. y?=w419:bool)
          n203 = call <vilib>:"WPI_EncoderGet.vi"("EncoderDevRef"=w435) -> ("Distance"=w440:dbl)  [unwired: 1 in, 9 out]
          n204 = call-poly <vilib>:"PID.vi"("output range"=cluster{"output high":dbl, "output low":dbl} {"output high"=1.0, "output low"=-1.0}, "PID gains"=w433, "process variable"=w439, "setpoint"=76.0) -> ("output"=w437:dbl)  [unwired: 3 in, 4 out]
          n205 = expression code="x/8"(w430) -> (w428:dbl)
          n206 = call-poly <vilib>:"PID.vi"("output range"=cluster{"output high":dbl, "output low":dbl} {"output high"=1.0, "output low"=-1.0}, "PID gains"=w433, "process variable"=w440, "setpoint"=388.0) -> ("output"=w442:dbl)  [unwired: 3 in, 4 out]
          n207 = Add(x=w429, y=w428) -> (x+y=w427:dbl)
          n208 = call <vilib>:"WPI_MotorControlSetOutput.vi"("Output"=w437, "MotorControlDevRef"=w431) -> ()  [unwired: 3 in, 7 out]
          n209 = call <vilib>:"WPI_RobotDriveMotors.vi"("RightSpeed"=w429, "LeftSpeed"=w427, "RobotDriveDevRef"=w421) -> ()  [unwired: 1 in, 8 out]
          n210 = call <vilib>:"WPI_MotorControlSetOutput.vi"("Output"=w442, "MotorControlDevRef"=w432) -> ()  [unwired: 3 in, 7 out]
          n211 = Select(t=i64 3, s=w419, f=w417) -> (s? t:f=w420:i64)
        }
        frame 3 {
          w462 = 0.0 ("LeftSpeed")
          # "x"
          # "open gripper"
          n212 = case shown="True" w458 {
            tunnel: w460 -> [w466 w470]
            tunnel: w459 -> [w465 _]
            frame False {
              n213 = call-poly <vilib>:"WPI_SolenoidSet.vi"("Value"=TRUE, "SolenoidDevRef"=w466) -> ()  [unwired: 1 in, 9 out]
              n214 = call-poly <vilib>:"WPI_SolenoidSet.vi"("Value"=FALSE, "SolenoidDevRef"=w465) -> ()  [unwired: 1 in, 9 out]
            }
            frame True {
              n215 = call-poly <vilib>:"WPI_SolenoidSet.vi"("Value"=TRUE, "SolenoidDevRef"=w470) -> ()  [unwired: 1 in, 9 out]
            }
          }
          n216 = call <vilib>:"WPI_MotorControlSetOutput.vi"("Output"=w462, "MotorControlDevRef"=w463) -> ()  [unwired: 3 in, 7 out]
          n217 = call <vilib>:"WPI_RobotDriveMotors.vi"("RightSpeed"=w462, "LeftSpeed"=w462, "RobotDriveDevRef"=w464) -> ()  [unwired: 1 in, 8 out]
          n218 = call <vilib>:"WPI_EncoderGet.vi"("EncoderDevRef"=w454) -> ("Distance"=w455:dbl)  [unwired: 1 in, 9 out]
          n219 = call-poly <vilib>:"PID.vi"("output range"=cluster{"output high":dbl, "output low":dbl} {"output high"=1.0, "output low"=-1.0}, "PID gains"=T16 {"proportional gain (Kc)"=-0.04, "integral time (Ti, min)"=0.0, "derivative time (Td, min)"=0.0}, "process variable"=w455, "setpoint"=76.0) -> ("output"=w452:dbl)  [unwired: 3 in, 4 out]
          n220 = call <vilib>:"WPI_MotorControlSetOutput.vi"("Output"=w452, "MotorControlDevRef"=w451) -> ()  [unwired: 3 in, 7 out]
          n221 = Wait (ms)(milliseconds to wait=u32 1500) -> ()  [unwired: 1 out]
        }
        frame 4 {
          w489 = 178.0 ("y")
          n222 = Less Or Equal?(x=w487, y=w489) -> (x <= y?=w490:bool)
          n223 = Less Or Equal?(x=w488, y=w489) -> (x <= y?=w491:bool)
          n224 = Subtract(x=w488, y=w487) -> (x-y=w486:dbl)
          n225 = case shown="True" w476 {
            tunnel: w475 -> [w500 w507]
            tunnel: w474 -> [w499 _]
            tunnel: w473 -> [_ w505]
            tunnel: [_ w503] -> w472
            frame False {
              n226 = call-poly <vilib>:"WPI_SolenoidSet.vi"("Value"=TRUE, "SolenoidDevRef"=w500) -> ()  [unwired: 1 in, 9 out]
              n227 = call-poly <vilib>:"WPI_SolenoidSet.vi"("Value"=FALSE, "SolenoidDevRef"=w499) -> ()  [unwired: 1 in, 9 out]
            }
            frame True {
              n228 = call-poly <vilib>:"WPI_SolenoidSet.vi"("Value"=TRUE, "SolenoidDevRef"=w507) -> ()  [unwired: 1 in, 9 out]
              n229 = call-poly <vilib>:"WPI_SolenoidSet.vi"("Value"=FALSE, "SolenoidDevRef"=w505) -> ("error out"=w503:errorcluster)  [unwired: 1 in, 8 out]
            }
          }
          n230 = And(x=w491, y=w490) -> ()  [unwired: 1 out]
          n231 = disable-structure shown="Disabled" {
            disable-tunnel: w486 -> [w509 _]
            disable-tunnel: w485 -> [w508 _]
            frame Disabled {
              w510 = -0.7 ("x")
              n232 = expression code="x/8"(w509) -> (w511:dbl)
              n233 = Add(x=w510, y=w511) -> (x+y=w512:dbl)
              n234 = call <vilib>:"WPI_RobotDriveMotors.vi"("RightSpeed"=w510, "LeftSpeed"=w512, "RobotDriveDevRef"=w508) -> ()  [unwired: 1 in, 8 out]
            }
            frame Enabled {
            }
          }
          n235 = flat-sequence {
            tunnel: w472 -> [w493]
            tunnel: [w493] -> w471
            frame #0 {
              n236 = Wait (ms)(milliseconds to wait=u32 750) -> ()  [unwired: 1 out]
            }
          }
          n237 = call <vilib>:"WPI_EncoderGet.vi"("EncoderDevRef"=w477) -> ("Distance"=w481:dbl)  [unwired: 1 in, 9 out]
          n238 = flat-sequence {
            tunnel: [w498] -> w492
            tunnel: w484 -> [w496]
            tunnel: w471 -> [_]
            frame #0 {
              n239 = Select(t=i64 5, s=TRUE, f=w496) -> (s? t:f=w498:i64)
            }
          }
          n240 = call-poly <vilib>:"PID.vi"("output range"=cluster{"output high":dbl, "output low":dbl} {"output high"=1.0, "output low"=-1.0}, "PID gains"=T16 {"proportional gain (Kc)"=-0.04, "integral time (Ti, min)"=0.0, "derivative time (Td, min)"=0.0}, "process variable"=w481, "setpoint"=76.0) -> ("output"=w483:dbl)  [unwired: 3 in, 4 out]
          n241 = call <vilib>:"WPI_MotorControlSetOutput.vi"("Output"=w483, "MotorControlDevRef"=w478) -> ()  [unwired: 3 in, 7 out]
        }
        frame 5 {
          w525 = 0.0 ("LeftSpeed")
          n242 = case shown="True" w524 {
            tunnel: w523 -> [w542 _]
            tunnel: w522 -> [w541 w546]
            frame False {
              n243 = call-poly <vilib>:"WPI_SolenoidSet.vi"("Value"=FALSE, "SolenoidDevRef"=w542) -> ()  [unwired: 1 in, 9 out]
              n244 = call-poly <vilib>:"WPI_SolenoidSet.vi"("Value"=TRUE, "SolenoidDevRef"=w541) -> ()  [unwired: 1 in, 9 out]
            }
            frame True {
              n245 = call-poly <vilib>:"WPI_SolenoidSet.vi"("Value"=FALSE, "SolenoidDevRef"=w546) -> ()  [unwired: 1 in, 9 out]
            }
          }
          n246 = call <vilib>:"WPI_RobotDriveMotors.vi"("RightSpeed"=w525, "LeftSpeed"=w525, "RobotDriveDevRef"=w526) -> ()  [unwired: 1 in, 8 out]
          n247 = call <vilib>:"WPI_EncoderGet.vi"("EncoderDevRef"=w515) -> ("Distance"=w519:dbl)  [unwired: 1 in, 9 out]
          n248 = disable-structure shown="Enabled" {
            disable-tunnel: w514 -> [w529 _]
            disable-tunnel: [w527 i64 6 ("t")] -> w513
            frame Disabled {
              n249 = First Call?() -> (First Call?: T/F=w536:bool)
              n250 = feedback #5() -> (w531:u32)  [unwired: 1 out]
              n251 = case shown="False" w536 {
                tunnel: [w538 w539] -> w533
                tunnel: w531 -> [w538 _]
                tunnel: [w537 w539] -> w532
                frame False {
                  n252 = Tick Count (ms)() -> (millisecond timer value=w537:u32)
                }
                frame True {
                  n253 = Tick Count (ms)() -> (millisecond timer value=w539:u32)
                }
              }
              n254 = feedback-in #5(w533) -> ()
              n255 = Subtract(x=w532, y=w533) -> (x-y=w534:u32)
              n256 = Greater?(x=w534, y=u32 1000) -> (0:w530:bool)
              n257 = Select(t=i64 6, s=w530, f=w529) -> (s? t:f=w527:i64)
            }
            frame Enabled {
            }
          }
          n258 = call-poly <vilib>:"PID.vi"("output range"=cluster{"output high":dbl, "output low":dbl} {"output high"=1.0, "output low"=-1.0}, "PID gains"=T16 {"proportional gain (Kc)"=-0.04, "integral time (Ti, min)"=0.0, "derivative time (Td, min)"=0.0}, "process variable"=w519, "setpoint"=76.0) -> ("output"=w521:dbl)  [unwired: 3 in, 4 out]
          n259 = call <vilib>:"WPI_MotorControlSetOutput.vi"("Output"=w521, "MotorControlDevRef"=w516) -> ()  [unwired: 3 in, 7 out]
        }
        frame 6 {
          w556 = T16 {"proportional gain (Kc)"=-0.04, "integral time (Ti, min)"=0.0, "derivative time (Td, min)"=0.0} ("PID gains")
          w551 = 504.0 ("setpoint")
          # "drive backwords five feet"
          n260 = case shown="True" w554 {
            tunnel: [TRUE w580] -> w552
            tunnel: w569 -> [_ w579]
            tunnel: w568 -> [_ w578]
            tunnel: [w573 w577] -> w567
            tunnel: [w573 w575] -> w566
            frame False {
              w573 = 0.0
            }
            frame True {
              w575 = -0.5 ("x")
              w581 = 118.0 ("y")
              n261 = Less?(x=w579, y=w581) -> (x < y?=w583:bool)
              n262 = Less?(x=w578, y=w581) -> (x < y?=w582:bool)
              n263 = Subtract(x=w579, y=w578) -> (x-y=w574:dbl)
              n264 = And(x=w583, y=w582) -> (x .and. y?=w580:bool)
              n265 = expression code="x/10"(w574) -> (w576:dbl)
              n266 = Add(x=w575, y=w576) -> (x+y=w577:dbl)
            }
          }
          n267 = call <vilib>:"WPI_EncoderGet.vi"("EncoderDevRef"=w560) -> ("Distance"=w548:dbl)  [unwired: 1 in, 9 out]
          n268 = call <vilib>:"WPI_EncoderGet.vi"("EncoderDevRef"=w555) -> ("Distance"=w550:dbl)  [unwired: 1 in, 9 out]
          n269 = call-poly <vilib>:"PID.vi"("output range"=cluster{"output high":dbl, "output low":dbl} {"output high"=1.0, "output low"=-1.0}, "PID gains"=w556, "process variable"=w548, "setpoint"=87.0) -> ("output"=w563:dbl)  [unwired: 3 in, 4 out]
          n270 = call-poly <vilib>:"PID.vi"("output range"=cluster{"output high":dbl, "output low":dbl} {"output high"=1.0, "output low"=-1.0}, "PID gains"=w556, "process variable"=w550, "setpoint"=w551) -> ("output"=w558:dbl)  [unwired: 3 in, 4 out]
          n271 = call <vilib>:"WPI_MotorControlSetOutput.vi"("Output"=w563, "MotorControlDevRef"=w561) -> ()  [unwired: 3 in, 7 out]
          n272 = Greater Or Equal?(x=w550, y=w551) -> (x >= y?=w547:bool)
          n273 = call <vilib>:"WPI_RobotDriveMotors.vi"("RightSpeed"=w566, "LeftSpeed"=w567, "RobotDriveDevRef"=w565) -> ()  [unwired: 1 in, 8 out]
          n274 = call <vilib>:"WPI_MotorControlSetOutput.vi"("Output"=w558, "MotorControlDevRef"=w557) -> ()  [unwired: 3 in, 7 out]
          n275 = And(x=w547, y=w552) -> (x .and. y?=w553:bool)
          n276 = Select(t=i64 7, s=w553, f=w564) -> (s? t:f=w571:i64)
        }
        frame 7 {
          w596 = 0.0 ("LeftSpeed")
          # "wait"
          n277 = case shown="True" w592 {
            tunnel: w594 -> [w600 w606]
            tunnel: w593 -> [w599 _]
            tunnel: w584 -> [_ w603]
            frame False {
              n278 = call-poly <vilib>:"WPI_SolenoidSet.vi"("Value"=TRUE, "SolenoidDevRef"=w600) -> ()  [unwired: 1 in, 9 out]
              n279 = call-poly <vilib>:"WPI_SolenoidSet.vi"("Value"=FALSE, "SolenoidDevRef"=w599) -> ()  [unwired: 1 in, 9 out]
            }
            frame True {
              n280 = call-poly <vilib>:"WPI_SolenoidSet.vi"("Value"=TRUE, "SolenoidDevRef"=w606) -> ()  [unwired: 1 in, 9 out]
              n281 = call-poly <vilib>:"WPI_SolenoidSet.vi"("Value"=FALSE, "SolenoidDevRef"=w603) -> ()  [unwired: 1 in, 9 out]
            }
          }
          n282 = call <vilib>:"WPI_MotorControlSetOutput.vi"("Output"=w596, "MotorControlDevRef"=w597) -> ()  [unwired: 3 in, 7 out]
          n283 = call <vilib>:"WPI_RobotDriveMotors.vi"("RightSpeed"=w596, "LeftSpeed"=w596, "RobotDriveDevRef"=w598) -> ()  [unwired: 1 in, 8 out]
          n284 = call <vilib>:"WPI_EncoderGet.vi"("EncoderDevRef"=w588) -> ("Distance"=w589:dbl)  [unwired: 1 in, 9 out]
          n285 = call-poly <vilib>:"PID.vi"("output range"=cluster{"output high":dbl, "output low":dbl} {"output high"=1.0, "output low"=-1.0}, "PID gains"=T16 {"proportional gain (Kc)"=-0.04, "integral time (Ti, min)"=0.0, "derivative time (Td, min)"=0.0}, "process variable"=w589, "setpoint"=87.0) -> ("output"=w586:dbl)  [unwired: 3 in, 4 out]
          n286 = call <vilib>:"WPI_MotorControlSetOutput.vi"("Output"=w586, "MotorControlDevRef"=w585) -> ()  [unwired: 3 in, 7 out]
        }
      }
    }
    frame 5 {
      # "drive forward 10 ft\nmove arm high goal w/ extender\nrelease tube\ndrive back 5 feet, move arm a little"
      n287 = case shown="3" w619 {
        selector: w619 -> [w629 w642 w670 _ w735 w757 w807 _]
        tunnel: [w630 w663 w673 u32 4 ("t") w744 w756 w814 u32 7 ("t")] -> w623
        tunnel: w622 -> [_ w658 w676 _ w739 _ w812 _]
        tunnel: w621 -> [_ w657 w675 _ w738 _ w811 _]
        tunnel: w620 -> [_ w652 w674 w717 w736 w769 w808 w840]
        tunnel: w618 -> [_ _ w684 w704 w729 w759 w804 w827]
        tunnel: w617 -> [_ _ w687 w707 w728 w758 w803 w830]
        tunnel: w616 -> [_ _ w688 _ _ _ w798 _]
        tunnel: w615 -> [_ _ w685 w716 _ _ w800 w839]
        tunnel: w614 -> [_ _ _ w713 w726 _ _ w836]
        tunnel: w613 -> [_ _ _ w712 w725 _ _ w835]
        tunnel: w612 -> [_ _ w669 w711 w727 w767 _ w834]
        tunnel: w611 -> [_ _ w668 _ _ w766 _ _]
        tunnel: w610 -> [_ _ w667 _ _ w765 _ _]
        tunnel: w609 -> [w625 _ _ _ _ _ _ _]
        tunnel: w608 -> [w624 _ _ _ _ _ _ _]
        tunnel: w607 -> [_ _ _ _ _ _ w797 _]
        frame 0, Default {
          # "reset encoders"
          n288 = disable-structure shown="Disabled" {
            disable-tunnel: [w633 _] -> _
            frame Disabled {
              n289 = feedback #6() -> (w638:u32)  [unwired: 1 out]
              n290 = case shown="False" {
                selector: _ -> [_ _]
                tunnel: [w640 w641] -> w636
                tunnel: w638 -> [w640 _]
                tunnel: [w639 w641] -> w637
                frame False {
                  n291 = Tick Count (ms)() -> (millisecond timer value=w639:u32)
                }
                frame True {
                  n292 = Tick Count (ms)() -> (millisecond timer value=w641:u32)
                }
              }
              n293 = feedback-in #6(w636) -> ()
              n294 = Subtract(x=w637, y=w636) -> (x-y=w635:u32)
              n295 = Greater?(x=w635, y=u32 3000) -> (0:w633:bool)
            }
            frame Enabled {
            }
          }
          n296 = First Call?() -> (First Call?: T/F=w626:bool)
          n297 = case shown="True" w626 {
            tunnel: w625 -> [_ w632]
            tunnel: w624 -> [_ w631]
            frame False {
            }
            frame True {
              n298 = call <vilib>:"WPI_EncoderReset.vi"("EncoderDevRef"=w631) -> ()  [unwired: 1 in, 10 out]
              n299 = call <vilib>:"WPI_EncoderReset.vi"("EncoderDevRef"=w632) -> ()  [unwired: 1 in, 10 out]
            }
          }
          n300 = Select(t=i64 1, s=TRUE, f=w629) -> (s? t:f=w630:i64)
        }
        frame 1 {
          w654 = 0.7 ("x")
          w659 = 182.0 ("y")
          # "drive forward 170 inches, advance in 1.5 seconds"
          n301 = Greater Or Equal?(x=w658, y=w659) -> (x >= y?=w661:bool)
          n302 = Greater Or Equal?(x=w657, y=w659) -> (x >= y?=w660:bool)
          n303 = Subtract(x=w658, y=w657) -> (x-y=w653:dbl)
          n304 = And(x=w661, y=w660) -> (x .and. y?=w646:bool)
          n305 = expression code="x/8"(w653) -> (w655:dbl)
          n306 = First Call?() -> (First Call?: T/F=w643:bool)
          n307 = Add(x=w654, y=w655) -> (x+y=w656:dbl)
          n308 = feedback #7() -> (w647:u32)  [unwired: 1 out]
          n309 = case shown="False" w643 {
            tunnel: [w665 w666] -> w649
            tunnel: w647 -> [w665 _]
            tunnel: [w664 w666] -> w648
            frame False {
              n310 = Tick Count (ms)() -> (millisecond timer value=w664:u32)
            }
            frame True {
              n311 = Tick Count (ms)() -> (millisecond timer value=w666:u32)
            }
          }
          n312 = feedback-in #7(w649) -> ()
          n313 = call <vilib>:"WPI_RobotDriveMotors.vi"("RightSpeed"=w654, "LeftSpeed"=w656, "RobotDriveDevRef"=w652) -> ()  [unwired: 1 in, 8 out]
          n314 = Subtract(x=w648, y=w649) -> (x-y=w650:u32)
          n315 = Greater?(x=w650, y=u32 1500) -> (0:w645:bool)
          n316 = Or(x=w645, y=w646) -> (x .or. y?=w644:bool)
          n317 = Select(t=i64 2, s=w644, f=w642) -> (s? t:f=w663:i64)
        }
        frame 2 {
          w686 = T16 {"proportional gain (Kc)"=-0.04, "integral time (Ti, min)"=0.0, "derivative time (Td, min)"=0.0} ("PID gains")
          w682 = 0.7 ("x")
          w679 = 182.0 ("y")
          # "drive 170 inches, move arm to high position, extend extender"
          n318 = case shown="True" w669 {
            tunnel: w668 -> [w699 w702]
            tunnel: w667 -> [w700 _]
            frame False {
              n319 = call-poly <vilib>:"WPI_SolenoidSet.vi"("Value"=TRUE, "SolenoidDevRef"=w699) -> ()  [unwired: 1 in, 9 out]
              n320 = call-poly <vilib>:"WPI_SolenoidSet.vi"("Value"=FALSE, "SolenoidDevRef"=w700) -> ()  [unwired: 1 in, 9 out]
            }
            frame True {
              n321 = call-poly <vilib>:"WPI_SolenoidSet.vi"("Value"=TRUE, "SolenoidDevRef"=w702) -> ()  [unwired: 1 in, 9 out]
            }
          }
          n322 = Greater Or Equal?(x=w676, y=w679) -> (x >= y?=w677:bool)
          n323 = Greater Or Equal?(x=w675, y=w679) -> (x >= y?=w678:bool)
          n324 = call <vilib>:"WPI_EncoderGet.vi"("EncoderDevRef"=w687) -> ("Distance"=w692:dbl)  [unwired: 1 in, 9 out]
          n325 = Subtract(x=w676, y=w675) -> (x-y=w683:dbl)
          n326 = And(x=w677, y=w678) -> (x .and. y?=w672:bool)
          n327 = call <vilib>:"WPI_EncoderGet.vi"("EncoderDevRef"=w688) -> ("Distance"=w693:dbl)  [unwired: 1 in, 9 out]
          n328 = call-poly <vilib>:"PID.vi"("output range"=cluster{"output high":dbl, "output low":dbl} {"output high"=1.0, "output low"=-1.0}, "PID gains"=w686, "process variable"=w692, "setpoint"=76.0) -> ("output"=w690:dbl)  [unwired: 3 in, 4 out]
          n329 = expression code="x/8"(w683) -> (w681:dbl)
          n330 = call-poly <vilib>:"PID.vi"("output range"=cluster{"output high":dbl, "output low":dbl} {"output high"=1.0, "output low"=-1.0}, "PID gains"=w686, "process variable"=w693, "setpoint"=388.0) -> ("output"=w695:dbl)  [unwired: 3 in, 4 out]
          n331 = Add(x=w682, y=w681) -> (x+y=w680:dbl)
          n332 = call <vilib>:"WPI_MotorControlSetOutput.vi"("Output"=w690, "MotorControlDevRef"=w684) -> ()  [unwired: 3 in, 7 out]
          n333 = call <vilib>:"WPI_RobotDriveMotors.vi"("RightSpeed"=w682, "LeftSpeed"=w680, "RobotDriveDevRef"=w674) -> ()  [unwired: 1 in, 8 out]
          n334 = call <vilib>:"WPI_MotorControlSetOutput.vi"("Output"=w695, "MotorControlDevRef"=w685) -> ()  [unwired: 3 in, 7 out]
          n335 = Select(t=i64 3, s=w672, f=w670) -> (s? t:f=w673:i64)
        }
        frame 3 {
          w715 = 0.0 ("LeftSpeed")
          # "stop, open gripper"
          n336 = case shown="True" w711 {
            tunnel: w713 -> [w719 w723]
            tunnel: w712 -> [w718 _]
            frame False {
              n337 = call-poly <vilib>:"WPI_SolenoidSet.vi"("Value"=TRUE, "SolenoidDevRef"=w719) -> ()  [unwired: 1 in, 9 out]
              n338 = call-poly <vilib>:"WPI_SolenoidSet.vi"("Value"=FALSE, "SolenoidDevRef"=w718) -> ()  [unwired: 1 in, 9 out]
            }
            frame True {
              n339 = call-poly <vilib>:"WPI_SolenoidSet.vi"("Value"=TRUE, "SolenoidDevRef"=w723) -> ()  [unwired: 1 in, 9 out]
            }
          }
          n340 = call <vilib>:"WPI_MotorControlSetOutput.vi"("Output"=w715, "MotorControlDevRef"=w716) -> ()  [unwired: 3 in, 7 out]
          n341 = call <vilib>:"WPI_RobotDriveMotors.vi"("RightSpeed"=w715, "LeftSpeed"=w715, "RobotDriveDevRef"=w717) -> ()  [unwired: 1 in, 8 out]
          n342 = call <vilib>:"WPI_EncoderGet.vi"("EncoderDevRef"=w707) -> ("Distance"=w708:dbl)  [unwired: 1 in, 9 out]
          n343 = call-poly <vilib>:"PID.vi"("output range"=cluster{"output high":dbl, "output low":dbl} {"output high"=1.0, "output low"=-1.0}, "PID gains"=T16 {"proportional gain (Kc)"=-0.04, "integral time (Ti, min)"=0.0, "derivative time (Td, min)"=0.0}, "process variable"=w708, "setpoint"=76.0) -> ("output"=w705:dbl)  [unwired: 3 in, 4 out]
          n344 = call <vilib>:"WPI_MotorControlSetOutput.vi"("Output"=w705, "MotorControlDevRef"=w704) -> ()  [unwired: 3 in, 7 out]
          n345 = Wait (ms)(milliseconds to wait=u32 1500) -> ()  [unwired: 1 out]
        }
        frame 4 {
          w740 = 182.0 ("y")
          # "keep gripper open"
          n346 = Less Or Equal?(x=w738, y=w740) -> (x <= y?=w741:bool)
          n347 = Less Or Equal?(x=w739, y=w740) -> (x <= y?=w742:bool)
          n348 = Subtract(x=w739, y=w738) -> (x-y=w737:dbl)
          n349 = case shown="True" w727 {
            tunnel: w726 -> [w746 w750]
            tunnel: w725 -> [w745 _]
            frame False {
              n350 = call-poly <vilib>:"WPI_SolenoidSet.vi"("Value"=TRUE, "SolenoidDevRef"=w746) -> ()  [unwired: 1 in, 9 out]
              n351 = call-poly <vilib>:"WPI_SolenoidSet.vi"("Value"=FALSE, "SolenoidDevRef"=w745) -> ()  [unwired: 1 in, 9 out]
            }
            frame True {
              n352 = call-poly <vilib>:"WPI_SolenoidSet.vi"("Value"=TRUE, "SolenoidDevRef"=w750) -> ()  [unwired: 1 in, 9 out]
            }
          }
          n353 = And(x=w742, y=w741) -> ()  [unwired: 1 out]
          n354 = disable-structure shown="Disabled" {
            disable-tunnel: w737 -> [w752 _]
            disable-tunnel: w736 -> [w751 _]
            frame Disabled {
              w753 = -0.7 ("x")
              n355 = expression code="x/8"(w752) -> (w754:dbl)
              n356 = Add(x=w753, y=w754) -> (x+y=w755:dbl)
              n357 = call <vilib>:"WPI_RobotDriveMotors.vi"("RightSpeed"=w753, "LeftSpeed"=w755, "RobotDriveDevRef"=w751) -> ()  [unwired: 1 in, 8 out]
            }
            frame Enabled {
            }
          }
          n358 = call <vilib>:"WPI_EncoderGet.vi"("EncoderDevRef"=w728) -> ("Distance"=w732:dbl)  [unwired: 1 in, 9 out]
          n359 = call-poly <vilib>:"PID.vi"("output range"=cluster{"output high":dbl, "output low":dbl} {"output high"=1.0, "output low"=-1.0}, "PID gains"=T16 {"proportional gain (Kc)"=-0.04, "integral time (Ti, min)"=0.0, "derivative time (Td, min)"=0.0}, "process variable"=w732, "setpoint"=76.0) -> ("output"=w734:dbl)  [unwired: 3 in, 4 out]
          n360 = Select(t=i64 5, s=TRUE, f=w735) -> (s? t:f=w744:i64)
          n361 = call <vilib>:"WPI_MotorControlSetOutput.vi"("Output"=w734, "MotorControlDevRef"=w729) -> ()  [unwired: 3 in, 7 out]
        }
        frame 5 {
          w768 = 0.0 ("LeftSpeed")
          # "bring extender in"
          n362 = case shown="True" w767 {
            tunnel: w766 -> [w785 _]
            tunnel: w765 -> [w784 w789]
            frame False {
              n363 = call-poly <vilib>:"WPI_SolenoidSet.vi"("Value"=FALSE, "SolenoidDevRef"=w785) -> ()  [unwired: 1 in, 9 out]
              n364 = call-poly <vilib>:"WPI_SolenoidSet.vi"("Value"=TRUE, "SolenoidDevRef"=w784) -> ()  [unwired: 1 in, 9 out]
            }
            frame True {
              n365 = call-poly <vilib>:"WPI_SolenoidSet.vi"("Value"=FALSE, "SolenoidDevRef"=w789) -> ()  [unwired: 1 in, 9 out]
            }
          }
          n366 = call <vilib>:"WPI_RobotDriveMotors.vi"("RightSpeed"=w768, "LeftSpeed"=w768, "RobotDriveDevRef"=w769) -> ()  [unwired: 1 in, 8 out]
          n367 = call <vilib>:"WPI_EncoderGet.vi"("EncoderDevRef"=w758) -> ("Distance"=w762:dbl)  [unwired: 1 in, 9 out]
          n368 = disable-structure shown="Disabled" {
            disable-tunnel: w757 -> [w772 _]
            disable-tunnel: [w770 i64 6 ("t")] -> w756
            frame Disabled {
              n369 = First Call?() -> (First Call?: T/F=w779:bool)
              n370 = feedback #8() -> (w774:u32)  [unwired: 1 out]
              n371 = case shown="False" w779 {
                tunnel: [w781 w782] -> w776
                tunnel: w774 -> [w781 _]
                tunnel: [w780 w782] -> w775
                frame False {
                  n372 = Tick Count (ms)() -> (millisecond timer value=w780:u32)
                }
                frame True {
                  n373 = Tick Count (ms)() -> (millisecond timer value=w782:u32)
                }
              }
              n374 = feedback-in #8(w776) -> ()
              n375 = Subtract(x=w775, y=w776) -> (x-y=w777:u32)
              n376 = Greater?(x=w777, y=u32 1000) -> (0:w773:bool)
              n377 = Select(t=i64 6, s=w773, f=w772) -> (s? t:f=w770:i64)
            }
            frame Enabled {
            }
          }
          n378 = call-poly <vilib>:"PID.vi"("output range"=cluster{"output high":dbl, "output low":dbl} {"output high"=1.0, "output low"=-1.0}, "PID gains"=T16 {"proportional gain (Kc)"=-0.04, "integral time (Ti, min)"=0.0, "derivative time (Td, min)"=0.0}, "process variable"=w762, "setpoint"=76.0) -> ("output"=w764:dbl)  [unwired: 3 in, 4 out]
          n379 = call <vilib>:"WPI_MotorControlSetOutput.vi"("Output"=w764, "MotorControlDevRef"=w759) -> ()  [unwired: 3 in, 7 out]
        }
        frame 6 {
          w799 = T16 {"proportional gain (Kc)"=-0.04, "integral time (Ti, min)"=0.0, "derivative time (Td, min)"=0.0} ("PID gains")
          w794 = 504.0 ("setpoint")
          # "drive backwords five feet"
          n380 = case shown="True" w797 {
            tunnel: [TRUE w823] -> w795
            tunnel: w812 -> [_ w822]
            tunnel: w811 -> [_ w821]
            tunnel: [w816 w820] -> w810
            tunnel: [w816 w818] -> w809
            frame False {
              w816 = 0.0
            }
            frame True {
              w818 = -0.5 ("x")
              w824 = 122.0 ("y")
              n381 = Less?(x=w822, y=w824) -> (x < y?=w826:bool)
              n382 = Less?(x=w821, y=w824) -> (x < y?=w825:bool)
              n383 = Subtract(x=w822, y=w821) -> (x-y=w817:dbl)
              n384 = And(x=w826, y=w825) -> (x .and. y?=w823:bool)
              n385 = expression code="x/10"(w817) -> (w819:dbl)
              n386 = Add(x=w818, y=w819) -> (x+y=w820:dbl)
            }
          }
          n387 = call <vilib>:"WPI_EncoderGet.vi"("EncoderDevRef"=w803) -> ("Distance"=w791:dbl)  [unwired: 1 in, 9 out]
          n388 = call <vilib>:"WPI_EncoderGet.vi"("EncoderDevRef"=w798) -> ("Distance"=w793:dbl)  [unwired: 1 in, 9 out]
          n389 = call-poly <vilib>:"PID.vi"("output range"=cluster{"output high":dbl, "output low":dbl} {"output high"=1.0, "output low"=-1.0}, "PID gains"=w799, "process variable"=w791, "setpoint"=87.0) -> ("output"=w806:dbl)  [unwired: 3 in, 4 out]
          n390 = call-poly <vilib>:"PID.vi"("output range"=cluster{"output high":dbl, "output low":dbl} {"output high"=1.0, "output low"=-1.0}, "PID gains"=w799, "process variable"=w793, "setpoint"=w794) -> ("output"=w801:dbl)  [unwired: 3 in, 4 out]
          n391 = call <vilib>:"WPI_MotorControlSetOutput.vi"("Output"=w806, "MotorControlDevRef"=w804) -> ()  [unwired: 3 in, 7 out]
          n392 = Greater Or Equal?(x=w793, y=w794) -> (x >= y?=w790:bool)
          n393 = call <vilib>:"WPI_RobotDriveMotors.vi"("RightSpeed"=w809, "LeftSpeed"=w810, "RobotDriveDevRef"=w808) -> ()  [unwired: 1 in, 8 out]
          n394 = call <vilib>:"WPI_MotorControlSetOutput.vi"("Output"=w801, "MotorControlDevRef"=w800) -> ()  [unwired: 3 in, 7 out]
          n395 = And(x=w790, y=w795) -> (x .and. y?=w796:bool)
          n396 = Select(t=i64 7, s=w796, f=w807) -> (s? t:f=w814:i64)
        }
        frame 7 {
          w838 = 0.0 ("LeftSpeed")
          # "wait"
          n397 = case shown="True" w834 {
            tunnel: w836 -> [w842 w846]
            tunnel: w835 -> [w841 _]
            frame False {
              n398 = call-poly <vilib>:"WPI_SolenoidSet.vi"("Value"=TRUE, "SolenoidDevRef"=w842) -> ()  [unwired: 1 in, 9 out]
              n399 = call-poly <vilib>:"WPI_SolenoidSet.vi"("Value"=FALSE, "SolenoidDevRef"=w841) -> ()  [unwired: 1 in, 9 out]
            }
            frame True {
              n400 = call-poly <vilib>:"WPI_SolenoidSet.vi"("Value"=TRUE, "SolenoidDevRef"=w846) -> ()  [unwired: 1 in, 9 out]
            }
          }
          n401 = call <vilib>:"WPI_MotorControlSetOutput.vi"("Output"=w838, "MotorControlDevRef"=w839) -> ()  [unwired: 3 in, 7 out]
          n402 = call <vilib>:"WPI_RobotDriveMotors.vi"("RightSpeed"=w838, "LeftSpeed"=w838, "RobotDriveDevRef"=w840) -> ()  [unwired: 1 in, 8 out]
          n403 = call <vilib>:"WPI_EncoderGet.vi"("EncoderDevRef"=w830) -> ("Distance"=w831:dbl)  [unwired: 1 in, 9 out]
          n404 = call-poly <vilib>:"PID.vi"("output range"=cluster{"output high":dbl, "output low":dbl} {"output high"=1.0, "output low"=-1.0}, "PID gains"=T16 {"proportional gain (Kc)"=-0.04, "integral time (Ti, min)"=0.0, "derivative time (Td, min)"=0.0}, "process variable"=w831, "setpoint"=87.0) -> ("output"=w828:dbl)  [unwired: 3 in, 4 out]
          n405 = call <vilib>:"WPI_MotorControlSetOutput.vi"("Output"=w828, "MotorControlDevRef"=w827) -> ()  [unwired: 3 in, 7 out]
        }
      }
    }
  }
  n406 = feedback-in #1(w37) -> ()
